vi "Reset Cursors.vi"(8 "Error In":errorcluster, 9 "x Cursor Ref Position":dbl format="%#_13g", 11 "Waveform Graph":refnum<vi>) -> (0 "error out":errorcluster)   [LabVIEW 2016]
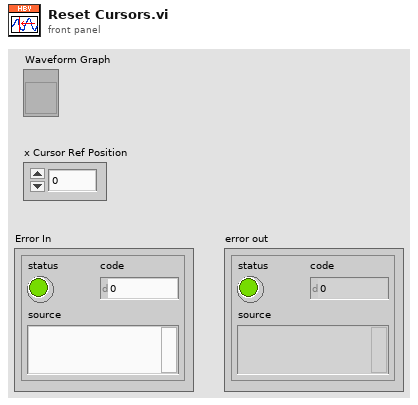
[diagram p1: front panel]
types:
  T1 = typedef "LVCursorListTypeDef.ctl" = cluster{"Name":string, "Color":u32, "Style":u8, "Point Style":u8, "Name Visible":bool, "Allow Drag":bool, "Cursor Mode":u32, "Plot":i32, "Index":i32, "Position":cluster{"X":dbl, "Y":dbl}, "X Scale":u32, "Y Scale":u32, "Watch Plots":i32[], "Watch All Plots":bool, "Plot Area":i32, "Label Offset":cluster{"X":dbl, "Y":dbl}}[]
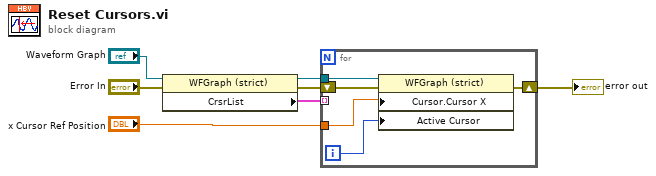
[diagram p0: block diagram]
diagram:
  n1 = property class="WFGraph (strict)"(reference="Waveform Graph", error in="Error In") -> (reference out=w2:refnum<vi>, error out=w4:errorcluster, "CrsrList"=w3:T1)
  n2 = for {
    tunnel: w3 -> [_] mode=indexing
    tunnel: w2 -> [w12]
    shift-right: [w10] -> w7
    shift-left: w4 -> [w9]
    tunnel: "x Cursor Ref Position" -> [w8]
    i -> [w11]
    n3 = property class="WFGraph (strict)"(reference=w12, error in=w9, "Cursor.Cursor X"=w8, "Active Cursor"=w11) -> (error out=w10:errorcluster)  [unwired: 1 out]
  }
  "error out" <- w7
